vi "subInitHW (niUSRP).vi"(0 "Tx Settings":T1={"USRP IP Address"="192.168.11.4", "IQ Sampling\nRate [S/sec]"=10000000.0, "Carrier Frequency [Hz]"=87000000.0, "Start Trigger Time"={"whole seconds"=0, "fractional seconds"=0.0}, "Per Device"=[]} {"Per Device"."gain" format="%#_6f"; "Carrier Frequency [Hz]" min=50000000.0 max=6000000000.0 step=1000.0 format="%#.15p"; "IQ Sampling\nRate [S/sec]" format="%#_6p"}, 5 "Rx Settings":T1={"USRP IP Address"="192.168.11.4", "IQ Sampling\nRate [S/sec]"=10000000.0, "Carrier Frequency [Hz]"=87000000.0, "Start Trigger Time"={"whole seconds"=0, "fractional seconds"=0.0}, "Per Device"=[]} {"Per Device"."gain" format="%#_6f"; "Carrier Frequency [Hz]" min=50000000.0 max=6000000000.0 step=1000.0 format="%#.15p"; "IQ Sampling\nRate [S/sec]" format="%#_6p"}, 11 "error in (no error)":errorcluster) -> (4 "Tx Settings (out)":T1={"USRP IP Address"="192.168.11.4", "IQ Sampling\nRate [S/sec]"=10000000.0, "Carrier Frequency [Hz]"=87000000.0, "Start Trigger Time"={"whole seconds"=0, "fractional seconds"=0.0}, "Per Device"=[]} {"Per Device"."gain" format="%#_6f"; "Carrier Frequency [Hz]" min=50000000.0 max=6000000000.0 step=1000.0 format="%#.15p"; "IQ Sampling\nRate [S/sec]" format="%#_6p"}, 6 "Rx Settings (out)":T1={"USRP IP Address"="192.168.11.4", "IQ Sampling\nRate [S/sec]"=10000000.0, "Carrier Frequency [Hz]"=87000000.0, "Start Trigger Time"={"whole seconds"=0, "fractional seconds"=0.0}, "Per Device"=[]} {"Per Device"."gain" format="%#_6f"; "Carrier Frequency [Hz]" min=50000000.0 max=6000000000.0 step=1000.0 format="%#.15p"; "IQ Sampling\nRate [S/sec]" format="%#_6p"}, 15 "error out":errorcluster)   [LabVIEW 2011]
uses:
  usrpHardwareSettings.ctl
  <instrlib>/niUSRP/niUSRP Timestamp.ctl
  <instrlib>/niUSRP/niUSRP Configure Time Start Trigger.vi
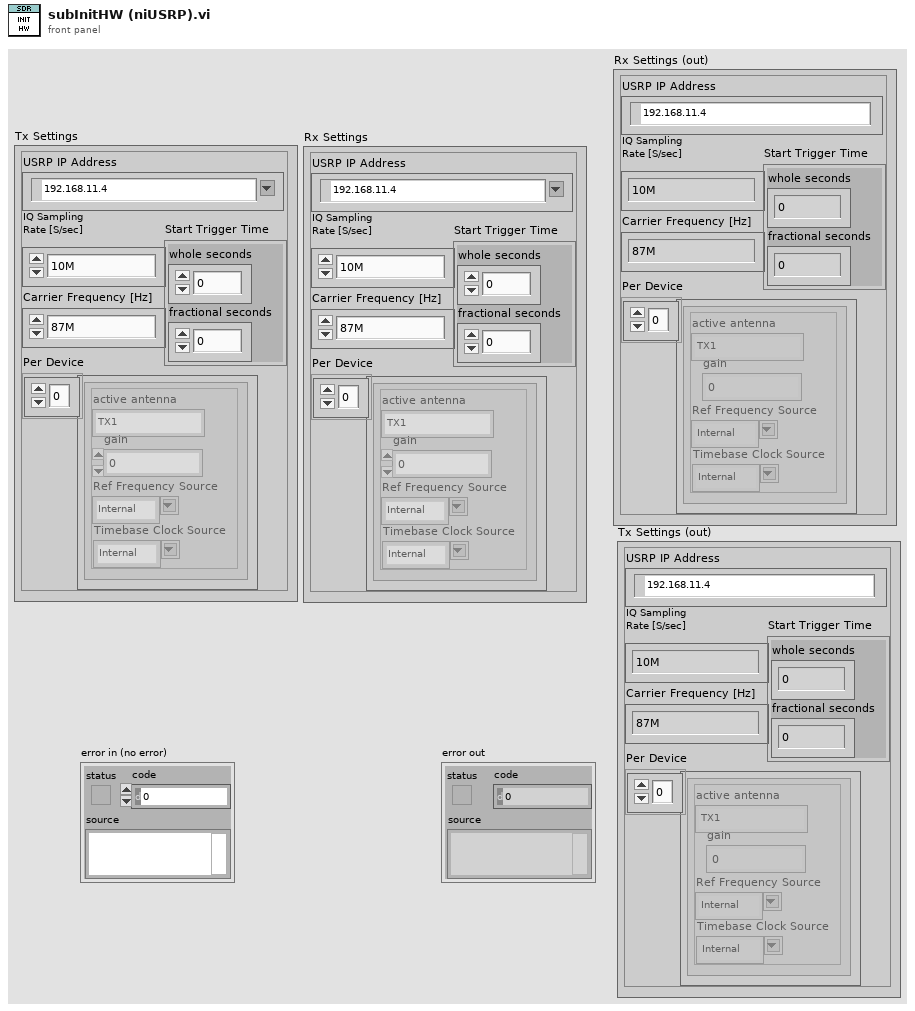
[diagram p1: front panel]
types:
  T1 = typedef "usrpHardwareSettings.ctl" = cluster{"USRP IP Address":refnum<k15>, "IQ Sampling\nRate [S/sec]":dbl, "Carrier Frequency [Hz]":dbl, "Start Trigger Time":T2, "Per Device":cluster{"active antenna":string, "gain":dbl, "Ref Frequency Source":string, "Timebase Clock Source":string}[]}
  T2 = typedef "niUSRP Timestamp.ctl" = cluster{"whole seconds":u64, "fractional seconds":dbl}
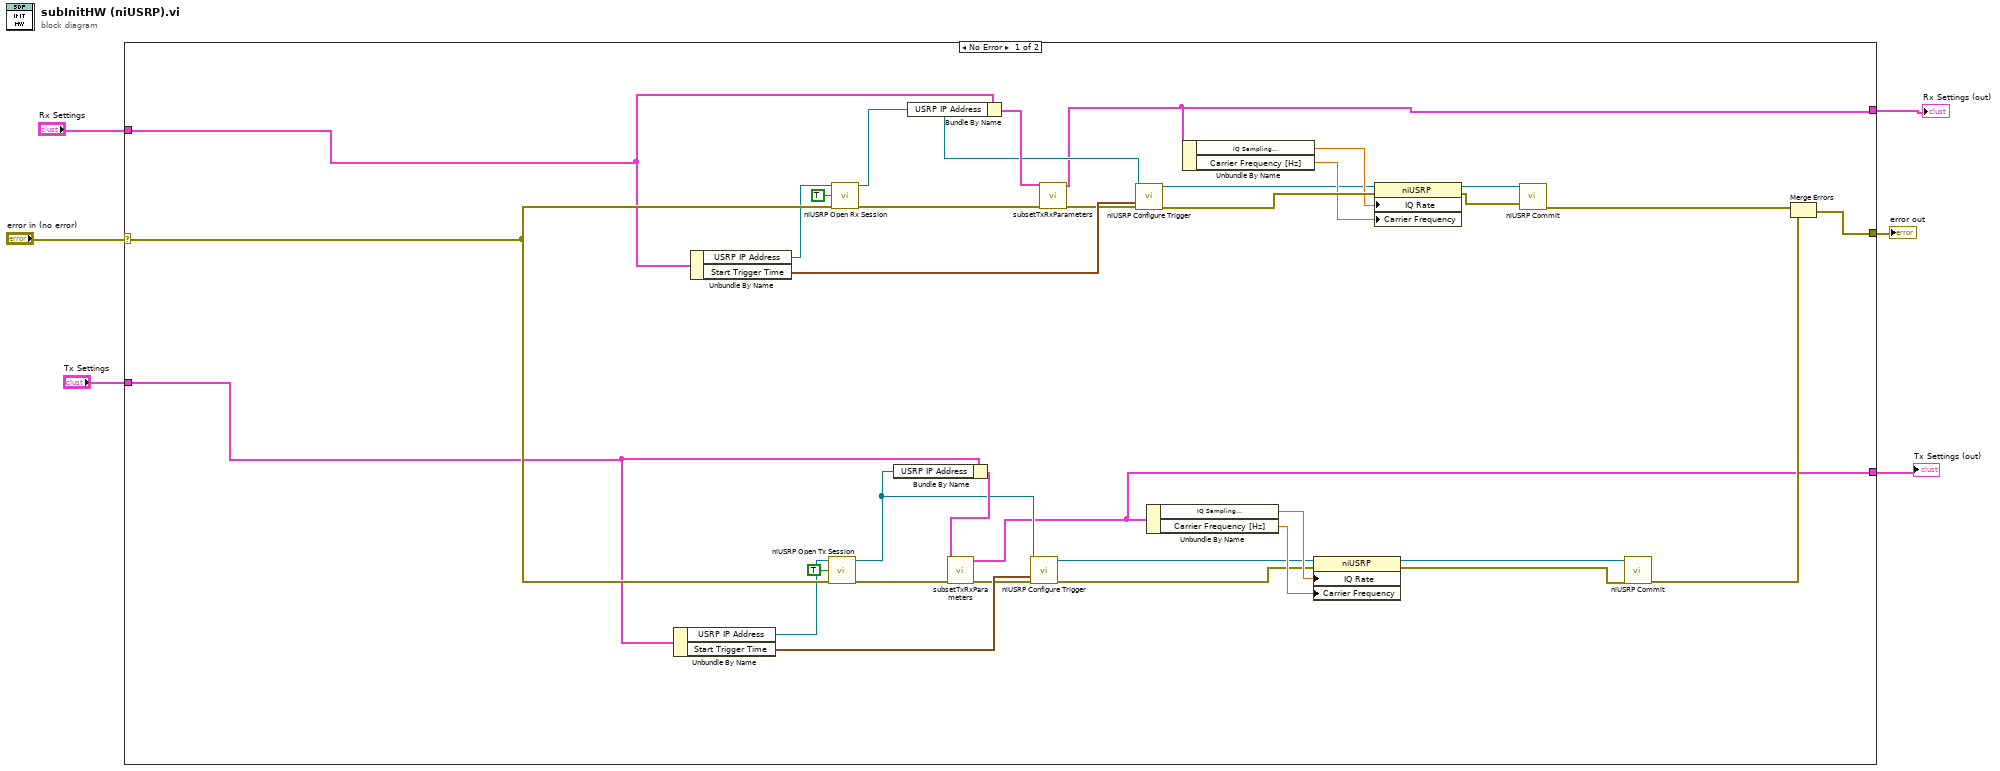
[diagram p0: block diagram]
diagram:
  n1 = case shown="No Error" "error in (no error)" {
    selector: "error in (no error)" -> [w40 w41]
    tunnel: [w39 w41] -> w5
    tunnel: [w9 _] -> w4
    tunnel: [w16 _] -> w3
    tunnel: "Rx Settings" -> [w15 _]
    tunnel: "Tx Settings" -> [w37 _]
    frame No Error {
      n2 = Unbundle By Name(w37) -> ("USRP IP Address"=w36:refnum<k15>, "Start Trigger Time"=w22:T2)
      n3 = Unbundle By Name(w15) -> ("USRP IP Address"=w38:refnum<k15>, "Start Trigger Time"=w35:T2)
      n4 = call <instrlib>:"niUSRP Open Tx Session.vi"("device names"=w36, "reset"=TRUE, "error in (no error)"=w40) -> ("session handle out"=w18:refnum<k15>, "error out"=w20:errorcluster)  [unwired: 11 in]
      n5 = call <instrlib>:"niUSRP Open Rx Session.vi"("device names"=w38, "reset"=TRUE, "error in (no error)"=w40) -> ("session handle out"=w11:refnum<k15>, "error out"=w14:errorcluster)  [unwired: 11 in]
      n6 = Bundle By Name(cluster=w37, "USRP IP Address"=w18) -> (w21:T1)
      n7 = Bundle By Name(cluster=w15, "USRP IP Address"=w11) -> (w13:T1)
      n8 = call "subsetTxRxParameters.vi"("Tx /Rx Settings"=w21, "error in (no error)"=w20) -> ("Tx /Rx  Settings (out)"=w16:T1, "error out"=w19:errorcluster)  [unwired: 12 in]
      n9 = call-poly <instrlib>:"niUSRP Configure Trigger.vi"("session handle"=w18, "start trigger time"=w22, "error in (no error)"=w19) -> ("session handle out"=w8:refnum<k15>, "error out"=w24:errorcluster)  [unwired: 11 in]
      n10 = call "subsetTxRxParameters.vi"("Tx /Rx Settings"=w13, "error in (no error)"=w14) -> ("Tx /Rx  Settings (out)"=w9:T1, "error out"=w12:errorcluster)  [unwired: 12 in]
      n11 = call-poly <instrlib>:"niUSRP Configure Trigger.vi"("session handle"=w11, "start trigger time"=w35, "error in (no error)"=w12) -> ("session handle out"=w7:refnum<k15>, "error out"=w30:errorcluster)  [unwired: 11 in]
      n12 = Unbundle By Name(w16) -> ("IQ Sampling\nRate [S/sec]"=w26:dbl, "Carrier Frequency [Hz]"=w25:dbl)
      n13 = Unbundle By Name(w9) -> ("IQ Sampling\nRate [S/sec]"=w28:dbl, "Carrier Frequency [Hz]"=w27:dbl)
      n14 = property class="niUSRP"(reference=w8, error in=w24, "IQ Rate"=w26, "Carrier Frequency"=w25) -> (reference out=w23:refnum<k15>, error out=w17:errorcluster)
      n15 = property class="niUSRP"(reference=w7, error in=w30, "IQ Rate"=w28, "Carrier Frequency"=w27) -> (reference out=w29:refnum<k15>, error out=w10:errorcluster)
      n16 = call <instrlib>:"niUSRP Commit.vi"("session handle"=w29, "error in (no error)"=w10) -> ("error out"=w32:errorcluster)  [unwired: 12 in, 1 out]
      n17 = call <instrlib>:"niUSRP Commit.vi"("session handle"=w23, "error in (no error)"=w17) -> ("error out"=w31:errorcluster)  [unwired: 12 in, 1 out]
      n18 = Merge Errors(w32, w31) -> (w39:errorcluster)
    }
    frame Error {
    }
  }
  "error out" <- w5
  "Rx Settings (out)" <- w4
  "Tx Settings (out)" <- w3
